vi "棋盘格搜索0元素.vi"(1 "无序一维坐标点":cluster{"X":sgl, "Y":sgl}[](array[cluster])=[{"X"=1412.6815, "Y"=3.6794338}, {"X"=950.6091, "Y"=7.2969584}, {"X"=1044.843, "Y"=8.55808}, {"X"=1048.5526, "Y"=6.4984}, {"X"=1137.2787, "Y"=6.285277}, {"X"=1139.5035, "Y"=6.383834}, {"X"=1229.4695, "Y"=6.128669}, {"X"=1233.7327, "Y"=5.9790673}, {"X"=1321.2677, "Y"=5.3170323}, {"X"=1326.042, "Y"=5.1197724}, {"X"=1418.9291, "Y"=5.099948}, {"X"=765.81134, "Y"=8.344691}, {"X"=769.6834, "Y"=8.466203}, {"X"=859.02246, "Y"=8.040275}, {"X"=862.6996, "Y"=7.9735875}, {"X"=579.4618, "Y"=10.38801}, {"X"=583.8774, "Y"=10.254913}, {"X"=950.7482, "Y"=10.59193}, {"X"=956.8515, "Y"=10.958951}, {"X"=1044.5778, "Y"=9.964842}, {"X"=1048.5502, "Y"=6.5010195}, {"X"=1137.2188, "Y"=9.72871}, {"X"=1140.8918, "Y"=9.898776}, {"X"=1229.8213, "Y"=9.607965}, {"X"=1233.8522, "Y"=9.771921}, {"X"=1321.432, "Y"=6.477976}, {"X"=1322.2452, "Y"=8.362788}, {"X"=1414.1876, "Y"=10.187137}, {"X"=1418.1567, "Y"=10.15385}, {"X"=1510.8711, "Y"=11.122694}, {"X"=394.15692, "Y"=12.698007}, {"X"=397.70276, "Y"=12.397687}, {"X"=486.81506, "Y"=11.80036}, {"X"=672.8406, "Y"=12.927005}, {"X"=676.3384, "Y"=12.897356}, {"X"=765.8697, "Y"=12.153455}, {"X"=769.6877, "Y"=11.942057}, {"X"=859.1302, "Y"=10.93324}, {"X"=209.12155, "Y"=15.971711}, {"X"=211.07715, "Y"=16.170942}, {"X"=301.63574, "Y"=15.61327}, {"X"=304.854, "Y"=17.051542}, {"X"=580.11304, "Y"=14.336995}, {"X"=583.01447, "Y"=14.092017}, {"X"=115.56893, "Y"=16.062284}, {"X"=120.1954, "Y"=17.73748}, {"X"=393.9527, "Y"=16.096884}, {"X"=397.5144, "Y"=15.868732}, {"X"=487.28784, "Y"=13.478283}, {"X"=490.1611, "Y"=13.438515}, {"X"=24.18013, "Y"=19.82086}, {"X"=28.127178, "Y"=19.778666}, {"X"=211.07715, "Y"=16.170942}, {"X"=301.23575, "Y"=17.503572}, {"X"=304.854, "Y"=17.051542}, {"X"=115.8368, "Y"=20.635664}, {"X"=120.1954, "Y"=17.73748}, {"X"=24.18013, "Y"=19.82086}, {"X"=28.127178, "Y"=19.778666}, {"X"=1045.7499, "Y"=99.26226}, {"X"=1049.2466, "Y"=98.93639}, {"X"=1138.3354, "Y"=98.90779}, {"X"=1142.3898, "Y"=98.86408}, {"X"=1231.339, "Y"=100.539635}, {"X"=1234.7195, "Y"=98.11695}, {"X"=1322.982, "Y"=98.044586}, {"X"=1327.0857, "Y"=98.04208}, {"X"=1415.0287, "Y"=97.80603}, {"X"=1419.0684, "Y"=98.0681}, {"X"=1505.3035, "Y"=96.962456}, {"X"=1512.1074, "Y"=97.130104}, {"X"=859.9964, "Y"=100.78096}, {"X"=863.6331, "Y"=100.47248}, {"X"=952.1462, "Y"=100.175026}, {"X"=957.658, "Y"=100.13256}, {"X"=580.6278, "Y"=103.213036}, {"X"=584.3985, "Y"=103.23712}, {"X"=673.80273, "Y"=102.282234}, {"X"=677.1538, "Y"=101.88441}, {"X"=767.1707, "Y"=101.07624}, {"X"=770.1185, "Y"=101.21626}, {"X"=1138.8663, "Y"=102.19401}, {"X"=1142.2152, "Y"=102.75242}, {"X"=1231.2098, "Y"=101.7738}, {"X"=1234.8201, "Y"=101.93511}, {"X"=1323.2035, "Y"=101.86018}, {"X"=1325.4602, "Y"=101.86024}, {"X"=1415.3267, "Y"=101.769135}, {"X"=1419.187, "Y"=102.09399}, {"X"=1506.1565, "Y"=102.658516}, {"X"=1508.5452, "Y"=102.83926}, {"X"=394.8409, "Y"=105.33422}, {"X"=397.97128, "Y"=106.54971}, {"X"=487.95963, "Y"=103.91474}, {"X"=489.4614, "Y"=104.11982}, {"X"=860.1312, "Y"=103.95015}, {"X"=863.5909, "Y"=103.99937}, {"X"=951.7162, "Y"=103.64365}, {"X"=957.8369, "Y"=103.65914}, {"X"=1045.9299, "Y"=102.832466}, {"X"=1049.6682, "Y"=102.73234}, {"X"=301.91907, "Y"=108.63288}, {"X"=305.55942, "Y"=106.17497}, {"X"=580.39777, "Y"=106.70424}, {"X"=673.86035, "Y"=105.7713}, {"X"=676.97003, "Y"=105.222305}, {"X"=767.33765, "Y"=105.11311}, {"X"=209.08888, "Y"=107.90821}, {"X"=213.45741, "Y"=108.1176}, {"X"=398.18994, "Y"=108.61662}, {"X"=487.44672, "Y"=107.1107}, {"X"=491.09204, "Y"=107.61974}, {"X"=584.32666, "Y"=106.886406}, {"X"=24.376457, "Y"=110.74549}, {"X"=29.008192, "Y"=112.00042}, {"X"=301.81976, "Y"=109.84095}, {"X"=305.561, "Y"=110.04465}, {"X"=117.142044, "Y"=113.09247}, {"X"=117.475876, "Y"=113.03857}, {"X"=209.28003, "Y"=111.63779}, {"X"=23.839958, "Y"=114.579}, {"X"=29.008192, "Y"=112.00042}, {"X"=1324.1991, "Y"=190.40904}, {"X"=1328.04, "Y"=190.72903}, {"X"=1415.9901, "Y"=190.3095}, {"X"=1420.0558, "Y"=189.9869}, {"X"=1507.3752, "Y"=193.75264}, {"X"=1512.9387, "Y"=189.73003}, {"X"=864.7421, "Y"=193.75208}, {"X"=952.7631, "Y"=193.2216}, {"X"=958.9441, "Y"=192.36739}, {"X"=1046.9897, "Y"=192.17368}, {"X"=1050.2294, "Y"=192.27582}, {"X"=1139.8049, "Y"=194.94722}, {"X"=1142.9745, "Y"=195.48999}, {"X"=767.46454, "Y"=194.17882}, {"X"=771.5019, "Y"=194.30862}, {"X"=861.0135, "Y"=193.35992}, {"X"=1231.742, "Y"=194.57672}, {"X"=1236.1552, "Y"=194.63904}, {"X"=1324.2634, "Y"=193.86778}, {"X"=1327.9126, "Y"=194.19914}, {"X"=1416.7396, "Y"=194.11032}, {"X"=1420.2114, "Y"=194.6422}, {"X"=1507.339, "Y"=194.16754}, {"X"=1512.0775, "Y"=194.51192}, {"X"=488.48718, "Y"=197.1191}, {"X"=491.92194, "Y"=197.1006}, {"X"=581.37964, "Y"=195.94873}, {"X"=584.89233, "Y"=195.9323}, {"X"=952.7631, "Y"=193.2216}, {"X"=958.8722, "Y"=195.93758}, {"X"=1046.9062, "Y"=195.63086}, {"X"=1050.1118, "Y"=193.37167}, {"X"=1139.8049, "Y"=194.94722}, {"X"=1142.9896, "Y"=195.51785}, {"X"=306.36182, "Y"=199.2471}, {"X"=395.10892, "Y"=197.99316}, {"X"=399.07867, "Y"=198.0709}, {"X"=678.3702, "Y"=198.62344}, {"X"=768.0162, "Y"=197.97568}, {"X"=771.06116, "Y"=198.24771}, {"X"=861.1216, "Y"=196.92929}, {"X"=864.5629, "Y"=197.49843}, {"X"=209.866, "Y"=200.47197}, {"X"=213.58813, "Y"=200.94618}, {"X"=302.78488, "Y"=198.96336}, {"X"=488.48718, "Y"=197.1191}, {"X"=492.23672, "Y"=200.02927}, {"X"=581.9015, "Y"=199.61447}, {"X"=585.0505, "Y"=199.66968}, {"X"=674.42084, "Y"=198.56363}, {"X"=25.285702, "Y"=202.90668}, {"X"=29.850668, "Y"=203.29842}, {"X"=117.47388, "Y"=204.86719}, {"X"=121.02383, "Y"=201.98978}, {"X"=306.60657, "Y"=202.69254}, {"X"=395.33936, "Y"=201.65161}, {"X"=398.54382, "Y"=201.6404}, {"X"=209.88214, "Y"=200.49939}, {"X"=213.58394, "Y"=200.949}, {"X"=25.198978, "Y"=206.81383}, {"X"=28.683458, "Y"=206.78719}, {"X"=117.47388, "Y"=204.86719}, {"X"=120.80801, "Y"=205.05066}, {"X"=1325.2671, "Y"=283.35147}, {"X"=1328.9977, "Y"=282.91864}, {"X"=1418.007, "Y"=282.4978}, {"X"=1421.0331, "Y"=282.4797}, {"X"=1509.221, "Y"=281.48706}, {"X"=1512.846, "Y"=282.29694}, {"X"=1047.7343, "Y"=285.08377}, {"X"=1051.6312, "Y"=285.14056}, {"X"=1141.0441, "Y"=284.36755}, {"X"=1144.0085, "Y"=284.42355}, {"X"=1232.844, "Y"=283.8645}, {"X"=1236.5856, "Y"=283.55615}, {"X"=768.8493, "Y"=287.1859}, {"X"=772.0435, "Y"=287.158}, {"X"=861.77344, "Y"=286.49255}, {"X"=865.5478, "Y"=286.81137}, {"X"=953.85864, "Y"=289.18365}, {"X"=959.21454, "Y"=285.9517}, {"X"=1325.3582, "Y"=286.68594}, {"X"=1329.0134, "Y"=286.73038}, {"X"=1417.3721, "Y"=286.148}, {"X"=1420.9364, "Y"=286.547}, {"X"=1509.0696, "Y"=286.48337}, {"X"=1512.7725, "Y"=286.69513}, {"X"=582.3613, "Y"=289.0204}, {"X"=586.0527, "Y"=289.16724}, {"X"=675.2951, "Y"=288.3512}, {"X"=679.0281, "Y"=287.99115}, {"X"=1047.8466, "Y"=288.6356}, {"X"=1051.0605, "Y"=289.00327}, {"X"=1140.4221, "Y"=287.8523}, {"X"=1144.0176, "Y"=287.8429}, {"X"=1236.9786, "Y"=287.531}, {"X"=396.21786, "Y"=291.33987}, {"X"=399.77203, "Y"=291.1318}, {"X"=489.97818, "Y"=290.03088}, {"X"=768.72845, "Y"=290.75858}, {"X"=862.06635, "Y"=289.9451}, {"X"=865.6694, "Y"=290.1604}, {"X"=953.85864, "Y"=289.18365}, {"X"=959.262, "Y"=289.76746}, {"X"=303.42657, "Y"=292.39053}, {"X"=306.9965, "Y"=292.31665}, {"X"=582.3937, "Y"=292.66464}, {"X"=585.84784, "Y"=292.1057}, {"X"=675.49225, "Y"=291.6714}, {"X"=678.7614, "Y"=292.08536}, {"X"=772.15295, "Y"=290.6915}, {"X"=118.36568, "Y"=294.27832}, {"X"=122.0356, "Y"=294.39282}, {"X"=396.16946, "Y"=294.61725}, {"X"=399.77203, "Y"=291.1318}, {"X"=489.8705, "Y"=294.09894}, {"X"=26.318064, "Y"=296.0619}, {"X"=29.029413, "Y"=296.98248}, {"X"=303.87878, "Y"=295.66165}, {"X"=307.0452, "Y"=295.67197}, {"X"=118.43474, "Y"=298.12512}, {"X"=121.986946, "Y"=297.7946}, {"X"=210.25739, "Y"=297.07492}, {"X"=214.33003, "Y"=296.81644}, {"X"=26.236132, "Y"=299.67172}, {"X"=29.051172, "Y"=297.44492}, {"X"=1509.8569, "Y"=375.06134}, {"X"=1515.014, "Y"=376.8497}, {"X"=1234.0524, "Y"=377.1514}, {"X"=1237.0068, "Y"=378.577}, {"X"=1326.3942, "Y"=376.00345}, {"X"=1329.9598, "Y"=375.93393}, {"X"=1418.275, "Y"=375.24207}, {"X"=1421.9374, "Y"=375.1909}, {"X"=954.8097, "Y"=378.36212}, {"X"=960.02106, "Y"=378.7047}, {"X"=1048.6476, "Y"=377.7871}, {"X"=1052.6216, "Y"=381.06326}, {"X"=1141.4268, "Y"=377.3096}, {"X"=1144.7307, "Y"=377.1711}, {"X"=1509.8569, "Y"=375.06134}, {"X"=1515.014, "Y"=376.8497}, {"X"=676.14905, "Y"=381.02945}, {"X"=769.40826, "Y"=380.4111}, {"X"=773.4843, "Y"=382.63983}, {"X"=862.42065, "Y"=379.4066}, {"X"=866.0779, "Y"=379.43088}, {"X"=1234.1095, "Y"=380.14008}, {"X"=1237.6244, "Y"=380.54337}, {"X"=1326.2516, "Y"=379.63504}, {"X"=1329.8422, "Y"=379.65314}, {"X"=1418.265, "Y"=378.85614}, {"X"=1421.9978, "Y"=379.1067}, {"X"=489.97784, "Y"=383.07867}, {"X"=493.81558, "Y"=382.8947}, {"X"=583.03766, "Y"=382.16656}, {"X"=586.826, "Y"=381.96048}, {"X"=954.73126, "Y"=382.2282}, {"X"=960.02106, "Y"=378.7047}, {"X"=1048.79, "Y"=381.73087}, {"X"=1052.6216, "Y"=381.06326}, {"X"=304.3866, "Y"=384.95547}, {"X"=307.9497, "Y"=385.10504}, {"X"=400.6453, "Y"=386.56058}, {"X"=676.1419, "Y"=384.64987}, {"X"=680.2898, "Y"=384.6469}, {"X"=769.6665, "Y"=383.59375}, {"X"=773.4509, "Y"=383.54562}, {"X"=862.7106, "Y"=383.15347}, {"X"=865.9845, "Y"=383.1695}, {"X"=122.703026, "Y"=387.3263}, {"X"=212.04758, "Y"=386.27716}, {"X"=215.01054, "Y"=386.17075}, {"X"=490.1799, "Y"=386.67773}, {"X"=493.9983, "Y"=386.97186}, {"X"=582.9337, "Y"=385.84512}, {"X"=587.5356, "Y"=385.06296}, {"X"=27.18197, "Y"=388.38385}, {"X"=27.18197, "Y"=388.38385}, {"X"=397.07806, "Y"=387.55035}, {"X"=211.91324, "Y"=389.84753}, {"X"=215.16852, "Y"=389.67154}, {"X"=26.72049, "Y"=391.7773}, {"X"=30.596046, "Y"=392.024}, {"X"=209.9042, "Y"=399.12137}, {"X"=1327.3544, "Y"=469.0647}, {"X"=1419.2324, "Y"=468.16718}, {"X"=1510.364, "Y"=467.17642}, {"X"=1514.4918, "Y"=470.6456}, {"X"=1049.9957, "Y"=471.0501}, {"X"=1052.8948, "Y"=470.93842}, {"X"=1142.4253, "Y"=470.17645}, {"X"=1145.9662, "Y"=470.30652}, {"X"=1235.0592, "Y"=469.96625}, {"X"=1238.565, "Y"=469.9739}, {"X"=864.0924, "Y"=472.51093}, {"X"=866.97833, "Y"=472.8782}, {"X"=955.69977, "Y"=471.45383}, {"X"=961.07306, "Y"=471.75146}, {"X"=1327.6859, "Y"=472.58783}, {"X"=1330.6233, "Y"=471.96988}, {"X"=1419.2172, "Y"=471.65576}, {"X"=1514.5454, "Y"=471.04782}, {"X"=680.64746, "Y"=474.37677}, {"X"=770.34247, "Y"=473.3417}, {"X"=774.00336, "Y"=473.83273}, {"X"=1049.3457, "Y"=474.62115}, {"X"=1142.9866, "Y"=473.95023}, {"X"=1145.7654, "Y"=473.9458}, {"X"=1234.9541, "Y"=473.04596}, {"X"=397.9174, "Y"=477.19165}, {"X"=402.21198, "Y"=477.09775}, {"X"=494.78082, "Y"=475.7434}, {"X"=584.2983, "Y"=474.8645}, {"X"=587.1738, "Y"=475.39746}, {"X"=864.05634, "Y"=476.47598}, {"X"=866.8885, "Y"=476.4903}, {"X"=955.8802, "Y"=475.2065}, {"X"=961.29596, "Y"=475.23154}, {"X"=212.9732, "Y"=479.274}, {"X"=216.23286, "Y"=479.20996}, {"X"=305.33755, "Y"=478.36325}, {"X"=308.86752, "Y"=478.19977}, {"X"=680.756, "Y"=477.63123}, {"X"=769.9319, "Y"=476.64694}, {"X"=773.70013, "Y"=476.8528}, {"X"=120.21636, "Y"=480.98227}, {"X"=123.844246, "Y"=480.48163}, {"X"=398.3618, "Y"=480.89243}, {"X"=401.6019, "Y"=480.75598}, {"X"=491.27213, "Y"=479.9286}, {"X"=494.78894, "Y"=479.69577}, {"X"=584.1824, "Y"=478.77087}, {"X"=587.6954, "Y"=478.91016}, {"X"=674.01056, "Y"=482.62982}, {"X"=212.80879, "Y"=482.5869}, {"X"=216.24107, "Y"=482.4923}, {"X"=305.47998, "Y"=481.54013}, {"X"=308.94867, "Y"=481.53357}, {"X"=31.690287, "Y"=484.7523}, {"X"=120.27868, "Y"=483.6429}, {"X"=123.6863, "Y"=483.62024}, {"X"=28.121384, "Y"=484.84103}, {"X"=1420.168, "Y"=559.44476}, {"X"=1423.1482, "Y"=559.8198}, {"X"=1511.3728, "Y"=558.7311}, {"X"=1514.719, "Y"=558.60486}, {"X"=1235.4536, "Y"=561.34454}, {"X"=1239.2461, "Y"=561.0861}, {"X"=1327.4503, "Y"=560.7745}, {"X"=1331.5977, "Y"=560.3296}, {"X"=1050.0205, "Y"=562.883}, {"X"=1053.6465, "Y"=563.0215}, {"X"=1142.638, "Y"=561.9079}, {"X"=1146.5131, "Y"=562.1473}, {"X"=772.0103, "Y"=565.13245}, {"X"=864.98785, "Y"=564.5342}, {"X"=864.98785, "Y"=564.5342}, {"X"=956.3751, "Y"=563.2659}, {"X"=962.3416, "Y"=563.8341}, {"X"=1511.809, "Y"=564.7066}, {"X"=588.1273, "Y"=567.27527}, {"X"=677.9531, "Y"=566.30536}, {"X"=681.8815, "Y"=565.8051}, {"X"=1329.0206, "Y"=566.27405}, {"X"=1329.0206, "Y"=566.27405}, {"X"=1420.063, "Y"=565.6257}, {"X"=1423.6278, "Y"=565.2837}, {"X"=1515.6139, "Y"=564.82184}, {"X"=396.0596, "Y"=569.9061}, {"X"=492.20886, "Y"=567.94684}, {"X"=495.66125, "Y"=568.28503}, {"X"=1050.3988, "Y"=568.6675}, {"X"=1053.7635, "Y"=568.8372}, {"X"=1143.1594, "Y"=567.572}, {"X"=1235.687, "Y"=567.51605}, {"X"=1239.5625, "Y"=566.922}, {"X"=213.8178, "Y"=570.6908}, {"X"=217.59773, "Y"=571.0198}, {"X"=306.02786, "Y"=570.01575}, {"X"=310.0028, "Y"=569.8299}, {"X"=864.40247, "Y"=570.1614}, {"X"=956.572, "Y"=569.1915}, {"X"=962.70074, "Y"=568.88965}, {"X"=32.6733, "Y"=572.6269}, {"X"=121.22974, "Y"=571.9324}, {"X"=678.23785, "Y"=572.22437}, {"X"=682.0419, "Y"=572.0976}, {"X"=771.42706, "Y"=571.2061}, {"X"=868.0665, "Y"=570.3193}, {"X"=492.17953, "Y"=573.8406}, {"X"=496.0425, "Y"=573.9344}, {"X"=588.7999, "Y"=572.8369}, {"X"=306.35614, "Y"=575.8801}, {"X"=309.8908, "Y"=575.51245}, {"X"=399.4254, "Y"=575.22363}, {"X"=121.18887, "Y"=577.85657}, {"X"=213.71536, "Y"=576.2731}, {"X"=217.2551, "Y"=576.7435}, {"X"=29.451935, "Y"=578.9594}, {"X"=1424.0056, "Y"=652.84735}, {"X"=1512.0708, "Y"=652.91266}, {"X"=1515.6927, "Y"=652.30774}, {"X"=1236.1508, "Y"=655.2158}, {"X"=1239.8197, "Y"=655.1497}, {"X"=1328.7433, "Y"=654.4055}, {"X"=1331.8887, "Y"=654.169}, {"X"=1420.2484, "Y"=653.17346}, {"X"=1051.1462, "Y"=657.3596}, {"X"=1054.7452, "Y"=657.3702}, {"X"=1143.0564, "Y"=657.12195}, {"X"=1147.328, "Y"=656.19324}, {"X"=1512.3021, "Y"=656.55066}, {"X"=1512.4271, "Y"=656.50757}, {"X"=868.06213, "Y"=658.3889}, {"X"=957.827, "Y"=658.16974}, {"X"=962.7932, "Y"=658.1109}, {"X"=1236.2236, "Y"=658.6412}, {"X"=1239.5663, "Y"=658.8228}, {"X"=1328.7885, "Y"=657.8645}, {"X"=1331.859, "Y"=657.7278}, {"X"=1423.7322, "Y"=657.41034}, {"X"=679.29376, "Y"=660.33417}, {"X"=772.2044, "Y"=662.99475}, {"X"=775.7194, "Y"=659.479}, {"X"=1051.1462, "Y"=657.3596}, {"X"=1054.7452, "Y"=657.3702}, {"X"=1142.9763, "Y"=657.51434}, {"X"=1147.4087, "Y"=659.037}, {"X"=493.21652, "Y"=662.3159}, {"X"=496.71637, "Y"=662.33325}, {"X"=589.6308, "Y"=661.3398}, {"X"=868.8922, "Y"=661.8618}, {"X"=957.336, "Y"=661.77264}, {"X"=961.2878, "Y"=663.0072}, {"X"=215.13858, "Y"=664.4556}, {"X"=217.96014, "Y"=664.7446}, {"X"=307.19785, "Y"=663.9552}, {"X"=311.07373, "Y"=664.37274}, {"X"=400.31244, "Y"=663.33}, {"X"=404.0007, "Y"=663.2761}, {"X"=586.37366, "Y"=665.0964}, {"X"=682.7313, "Y"=663.8328}, {"X"=772.2044, "Y"=662.99475}, {"X"=775.2198, "Y"=663.5096}, {"X"=30.386137, "Y"=666.41254}, {"X"=33.78909, "Y"=666.9363}, {"X"=122.40613, "Y"=665.84503}, {"X"=126.02608, "Y"=665.8279}, {"X"=492.90775, "Y"=665.8436}, {"X"=496.92422, "Y"=665.8403}, {"X"=214.90646, "Y"=668.46643}, {"X"=218.53204, "Y"=668.5923}, {"X"=307.47598, "Y"=667.53406}, {"X"=311.1581, "Y"=667.7079}, {"X"=403.96774, "Y"=666.58673}, {"X"=30.956583, "Y"=670.09735}, {"X"=31.453695, "Y"=670.0807}, {"X"=122.94276, "Y"=669.6548}, {"X"=125.77965, "Y"=669.294}, {"X"=1512.6708, "Y"=744.44354}, {"X"=1516.6038, "Y"=744.8743}, {"X"=1332.8044, "Y"=746.6566}, {"X"=1421.0765, "Y"=745.85065}, {"X"=1424.6377, "Y"=749.5571}, {"X"=1145.8118, "Y"=748.033}, {"X"=1146.9818, "Y"=748.2303}, {"X"=1236.9733, "Y"=748.09424}, {"X"=1236.9733, "Y"=748.09424}, {"X"=1512.4379, "Y"=748.0738}, {"X"=1516.5994, "Y"=748.53796}, {"X"=957.71515, "Y"=751.041}, {"X"=963.9972, "Y"=751.08954}, {"X"=1051.8019, "Y"=749.85675}, {"X"=1055.163, "Y"=749.92584}, {"X"=1332.627, "Y"=750.5142}, {"X"=1420.7009, "Y"=749.6165}, {"X"=1424.658, "Y"=749.5828}, {"X"=773.14355, "Y"=752.3674}, {"X"=866.12976, "Y"=751.4759}, {"X"=868.864, "Y"=754.5674}, {"X"=1144.3915, "Y"=752.5427}, {"X"=1147.6367, "Y"=752.30023}, {"X"=1237.0159, "Y"=751.5042}, {"X"=494.73883, "Y"=755.6712}, {"X"=497.8763, "Y"=755.1298}, {"X"=587.28986, "Y"=754.1544}, {"X"=679.9945, "Y"=753.2988}, {"X"=683.91077, "Y"=753.28455}, {"X"=957.874, "Y"=752.513}, {"X"=963.9972, "Y"=751.08954}, {"X"=1051.715, "Y"=752.9354}, {"X"=1055.2142, "Y"=753.10297}, {"X"=308.51486, "Y"=756.83453}, {"X"=311.88177, "Y"=756.9832}, {"X"=404.83005, "Y"=755.91406}, {"X"=772.84546, "Y"=755.67035}, {"X"=776.7339, "Y"=756.0081}, {"X"=868.2573, "Y"=755.0738}, {"X"=31.860968, "Y"=759.42645}, {"X"=35.618187, "Y"=759.91064}, {"X"=123.8723, "Y"=758.613}, {"X"=125.50653, "Y"=758.1765}, {"X"=216.27132, "Y"=757.9219}, {"X"=219.32713, "Y"=757.7127}, {"X"=497.8763, "Y"=755.1298}, {"X"=587.0371, "Y"=757.8683}, {"X"=590.6328, "Y"=757.74884}, {"X"=680.9836, "Y"=757.37994}, {"X"=309.1065, "Y"=760.28265}, {"X"=312.00598, "Y"=760.57916}, {"X"=404.73682, "Y"=759.76105}, {"X"=494.2343, "Y"=759.09515}, {"X"=1053.7183, "Y"=759.52075}, {"X"=32.036686, "Y"=762.72076}, {"X"=123.82045, "Y"=762.20496}, {"X"=127.40294, "Y"=762.11786}, {"X"=216.3088, "Y"=761.10406}, {"X"=219.51328, "Y"=760.9907}, {"X"=1512.7866, "Y"=836.7208}, {"X"=1516.1836, "Y"=836.706}, {"X"=1421.265, "Y"=838.0971}, {"X"=1237.2886, "Y"=840.30884}, {"X"=1240.8717, "Y"=840.2423}, {"X"=1516.0099, "Y"=840.84064}, {"X"=1052.3063, "Y"=842.35706}, {"X"=1055.8276, "Y"=842.0459}, {"X"=1144.8585, "Y"=841.3377}, {"X"=1421.244, "Y"=842.0497}, {"X"=775.316, "Y"=845.4439}, {"X"=866.7553, "Y"=843.96124}, {"X"=870.1111, "Y"=844.3156}, {"X"=966.4094, "Y"=845.16437}, {"X"=1148.0193, "Y"=844.9224}, {"X"=1237.1177, "Y"=843.7787}, {"X"=1240.814, "Y"=843.8384}, {"X"=1329.8593, "Y"=842.6638}, {"X"=1333.1106, "Y"=842.70825}, {"X"=588.2757, "Y"=846.72455}, {"X"=591.5033, "Y"=847.0653}, {"X"=681.00464, "Y"=846.18243}, {"X"=685.01025, "Y"=846.3228}, {"X"=774.0265, "Y"=845.37006}, {"X"=1052.2452, "Y"=845.84656}, {"X"=1055.5713, "Y"=845.9697}, {"X"=402.46408, "Y"=848.4553}, {"X"=405.85208, "Y"=849.1168}, {"X"=494.95795, "Y"=848.1302}, {"X"=498.768, "Y"=848.0817}, {"X"=863.88965, "Y"=845.8309}, {"X"=870.37415, "Y"=844.3211}, {"X"=958.74976, "Y"=846.77563}, {"X"=125.33506, "Y"=850.9014}, {"X"=128.75377, "Y"=851.14294}, {"X"=217.27446, "Y"=850.38837}, {"X"=309.9121, "Y"=849.8526}, {"X"=313.24408, "Y"=852.8987}, {"X"=587.80383, "Y"=850.5033}, {"X"=591.61615, "Y"=850.7564}, {"X"=681.3442, "Y"=849.82886}, {"X"=684.9827, "Y"=847.42126}, {"X"=33.159054, "Y"=852.04767}, {"X"=402.47308, "Y"=852.20996}, {"X"=405.83694, "Y"=852.06805}, {"X"=495.41132, "Y"=851.6362}, {"X"=498.69678, "Y"=851.55646}, {"X"=125.36255, "Y"=854.8094}, {"X"=128.62521, "Y"=853.93445}, {"X"=217.24501, "Y"=853.59094}, {"X"=221.00249, "Y"=854.06195}, {"X"=309.84454, "Y"=852.7346}, {"X"=313.24408, "Y"=852.8987}, {"X"=33.18453, "Y"=853.3919}, {"X"=1094.8916, "Y"=879.7679}, {"X"=1326.8314, "Y"=920.89703}, {"X"=1324.2201, "Y"=923.777}, {"X"=1325.2799, "Y"=923.7304}, {"X"=1513.0775, "Y"=929.07574}, {"X"=1516.8359, "Y"=928.95483}, {"X"=1421.9668, "Y"=930.1851}, {"X"=1425.1039, "Y"=930.08386}, {"X"=1237.4916, "Y"=933.0584}, {"X"=1240.8352, "Y"=932.4593}, {"X"=1331.0498, "Y"=931.4504}, {"X"=1331.0498, "Y"=931.4504}, {"X"=1512.8682, "Y"=932.8561}, {"X"=1516.886, "Y"=932.69073}, {"X"=1053.2501, "Y"=934.4577}, {"X"=1053.2501, "Y"=934.4577}, {"X"=1145.7811, "Y"=934.0479}, {"X"=1149.4984, "Y"=933.73804}, {"X"=1421.3748, "Y"=933.98804}, {"X"=1424.8423, "Y"=934.2104}, {"X"=867.4395, "Y"=937.1504}, {"X"=870.9637, "Y"=936.9113}, {"X"=959.7388, "Y"=935.8997}, {"X"=965.13367, "Y"=935.7838}, {"X"=1237.4745, "Y"=935.89185}, {"X"=1241.134, "Y"=935.9662}, {"X"=1330.0884, "Y"=934.9351}, {"X"=1333.5903, "Y"=935.0333}, {"X"=682.15985, "Y"=938.4487}, {"X"=685.06586, "Y"=938.4208}, {"X"=774.95917, "Y"=938.17334}, {"X"=778.5676, "Y"=938.227}, {"X"=1053.1005, "Y"=937.9979}, {"X"=1056.5786, "Y"=937.8953}, {"X"=1145.3656, "Y"=937.22943}, {"X"=1148.7098, "Y"=937.257}, {"X"=403.44504, "Y"=941.33777}, {"X"=406.92322, "Y"=940.8044}, {"X"=496.3331, "Y"=941.0075}, {"X"=499.9358, "Y"=940.97577}, {"X"=589.3127, "Y"=939.8238}, {"X"=867.4395, "Y"=937.1504}, {"X"=870.9637, "Y"=936.9113}, {"X"=959.3603, "Y"=939.2864}, {"X"=965.25543, "Y"=939.3708}, {"X"=222.5551, "Y"=942.39026}, {"X"=311.01688, "Y"=942.26483}, {"X"=314.80524, "Y"=943.13434}, {"X"=682.1386, "Y"=942.0657}, {"X"=685.58167, "Y"=942.0178}, {"X"=775.2412, "Y"=939.3993}, {"X"=778.5166, "Y"=941.0647}, {"X"=34.832672, "Y"=943.8151}, {"X"=34.832672, "Y"=943.8151}, {"X"=126.3559, "Y"=943.4925}, {"X"=130.02597, "Y"=943.2728}, {"X"=496.45908, "Y"=944.1266}, {"X"=499.9358, "Y"=940.97577}, {"X"=589.3983, "Y"=943.6146}, {"X"=592.84216, "Y"=941.2381}, {"X"=218.91013, "Y"=946.0248}, {"X"=222.81172, "Y"=945.8305}, {"X"=311.21887, "Y"=945.63025}, {"X"=314.0045, "Y"=945.7016}, {"X"=403.43817, "Y"=944.6669}, {"X"=407.33734, "Y"=944.66846}, {"X"=34.753956, "Y"=947.16754}, {"X"=37.952045, "Y"=945.3175}, {"X"=1513.1074, "Y"=1020.53687}, {"X"=1516.7944, "Y"=1020.3726}, {"X"=1422.1199, "Y"=1022.3085}, {"X"=1422.4272, "Y"=1022.35815}, {"X"=1237.7603, "Y"=1025.2195}, {"X"=1241.5918, "Y"=1024.5043}, {"X"=1330.0405, "Y"=1023.4761}, {"X"=1333.5803, "Y"=1023.4029}, {"X"=1512.2899, "Y"=1024.6274}, {"X"=1516.7074, "Y"=1024.4958}, {"X"=1053.4192, "Y"=1027.228}, {"X"=1057.2833, "Y"=1027.4166}, {"X"=1146.0155, "Y"=1026.057}, {"X"=1149.5197, "Y"=1026.0944}, {"X"=1422.1165, "Y"=1025.9506}, {"X"=1425.0371, "Y"=1025.8577}, {"X"=871.8444, "Y"=1029.0967}, {"X"=959.8629, "Y"=1027.9442}, {"X"=965.6788, "Y"=1027.915}, {"X"=1237.7603, "Y"=1025.2195}, {"X"=1241.622, "Y"=1028.4213}, {"X"=1330.1205, "Y"=1026.9482}, {"X"=1333.6062, "Y"=1027.1625}, {"X"=682.9343, "Y"=1031.4572}, {"X"=686.32434, "Y"=1030.9644}, {"X"=775.43744, "Y"=1030.3405}, {"X"=779.281, "Y"=1030.3405}, {"X"=868.21136, "Y"=1029.3007}, {"X"=1053.4773, "Y"=1030.0444}, {"X"=1057.2833, "Y"=1027.4166}, {"X"=1146.203, "Y"=1029.6053}, {"X"=1149.5355, "Y"=1026.4617}, {"X"=497.30618, "Y"=1033.2229}, {"X"=500.91095, "Y"=1033.2767}, {"X"=590.36127, "Y"=1032.0253}, {"X"=593.9072, "Y"=1031.889}, {"X"=959.7527, "Y"=1031.7665}, {"X"=966.0734, "Y"=1031.222}, {"X"=220.08049, "Y"=1035.1736}, {"X"=223.77623, "Y"=1035.241}, {"X"=312.41544, "Y"=1034.2931}, {"X"=315.8206, "Y"=1034.3982}, {"X"=405.34964, "Y"=1033.7988}, {"X"=408.60822, "Y"=1033.7543}, {"X"=682.841, "Y"=1034.1649}, {"X"=682.841, "Y"=1034.1649}, {"X"=776.06824, "Y"=1033.6057}, {"X"=778.93896, "Y"=1033.6743}, {"X"=868.1692, "Y"=1032.6964}, {"X"=872.0014, "Y"=1032.8055}, {"X"=36.842037, "Y"=1035.9076}, {"X"=39.936604, "Y"=1035.942}, {"X"=128.4923, "Y"=1035.3223}, {"X"=131.72397, "Y"=1035.3107}, {"X"=497.30618, "Y"=1033.2229}, {"X"=501.04752, "Y"=1036.593}, {"X"=589.87683, "Y"=1035.6193}, {"X"=593.91644, "Y"=1035.6195}, {"X"=220.08049, "Y"=1035.1736}, {"X"=223.65102, "Y"=1038.0187}, {"X"=312.88974, "Y"=1037.5582}, {"X"=315.66324, "Y"=1035.3694}, {"X"=405.17947, "Y"=1037.0765}, {"X"=36.871353, "Y"=1039.5012}, {"X"=40.06816, "Y"=1039.0924}, {"X"=128.34323, "Y"=1039.046}, {"X"=131.75531, "Y"=1039.057}, {"X"=313.3858, "Y"=1095.004}, {"X"=316.9034, "Y"=1099.374}, {"X"=1517.0452, "Y"=1112.1788}, {"X"=1330.4326, "Y"=1115.1825}, {"X"=1333.8274, "Y"=1115.1122}, {"X"=1421.7859, "Y"=1113.9792}, {"X"=1425.6499, "Y"=1113.939}, {"X"=1238.3629, "Y"=1116.9702}, {"X"=1242.0442, "Y"=1116.4863}, {"X"=1513.075, "Y"=1116.5619}, {"X"=1516.7253, "Y"=1116.6143}, {"X"=1053.9915, "Y"=1119.3153}, {"X"=1057.8392, "Y"=1119.2094}, {"X"=1146.4037, "Y"=1117.9922}, {"X"=1149.7257, "Y"=1118.2214}, {"X"=1421.878, "Y"=1117.6423}, {"X"=1425.1816, "Y"=1117.8027}, {"X"=960.61615, "Y"=1120.3813}, {"X"=966.5916, "Y"=1123.5236}, {"X"=1238.2561, "Y"=1119.9944}, {"X"=1241.798, "Y"=1120.231}, {"X"=777.1195, "Y"=1122.3763}, {"X"=779.82605, "Y"=1122.7509}, {"X"=869.13324, "Y"=1124.7325}, {"X"=1053.9915, "Y"=1119.3153}, {"X"=1057.8392, "Y"=1119.2094}, {"X"=1146.2975, "Y"=1121.5195}, {"X"=1149.6943, "Y"=1121.6158}, {"X"=498.38565, "Y"=1125.3086}, {"X"=502.0334, "Y"=1125.106}, {"X"=591.2226, "Y"=1124.0642}, {"X"=594.78864, "Y"=1123.7322}, {"X"=684.0514, "Y"=1126.7501}, {"X"=960.99854, "Y"=1123.7999}, {"X"=966.5531, "Y"=1123.76}, {"X"=130.10886, "Y"=1127.1348}, {"X"=133.22865, "Y"=1127.1709}, {"X"=221.75378, "Y"=1127.1466}, {"X"=225.48451, "Y"=1127.055}, {"X"=313.80075, "Y"=1126.9071}, {"X"=317.21503, "Y"=1126.3654}, {"X"=406.46625, "Y"=1128.915}, {"X"=409.8158, "Y"=1129.1194}, {"X"=687.5572, "Y"=1127.0116}, {"X"=776.7782, "Y"=1125.7067}, {"X"=780.0457, "Y"=1125.8667}, {"X"=869.13324, "Y"=1124.7325}, {"X"=37.945602, "Y"=1127.3896}, {"X"=41.87246, "Y"=1127.2628}, {"X"=499.2134, "Y"=1128.6807}, {"X"=502.0334, "Y"=1125.106}, {"X"=591.24805, "Y"=1127.5718}, {"X"=594.9117, "Y"=1127.5956}, {"X"=221.83293, "Y"=1130.5206}, {"X"=225.48451, "Y"=1127.055}, {"X"=313.7707, "Y"=1129.5864}, {"X"=317.70578, "Y"=1129.7416}, {"X"=406.46625, "Y"=1128.915}, {"X"=409.8158, "Y"=1129.1194}, {"X"=38.267227, "Y"=1131.0507}, {"X"=41.550556, "Y"=1131.6764}, {"X"=133.1631, "Y"=1130.7614}]) -> (0 "数值输入控件":i32)   [LabVIEW 2014]
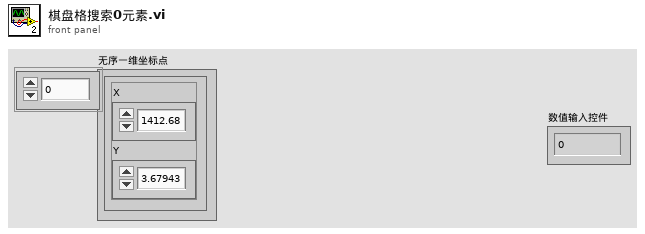
[diagram p1: front panel]
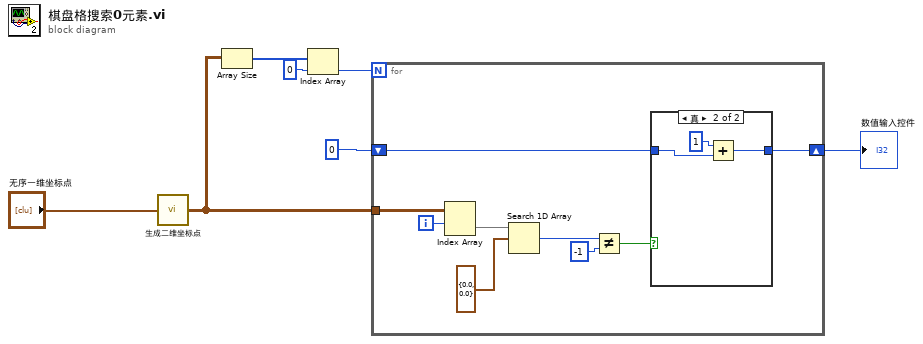
[diagram p0: block diagram]
diagram:
  n1 = call "生成二维坐标点.vi"("输入无序一维坐标点"="无序一维坐标点") -> ("输出有序二维坐标点"=w7:cluster{"X":sgl, "Y":sgl}[][])
  n2 = Array Size(array=w7) -> (size(s)=w6:i32[])
  n3 = Index Array(array=w6, index=0 ("索引")) -> (element=w4:i32)
  n4 = for {
    N: w4 -> [_]
    tunnel: w7 -> [w16]
    shift-right: [w12] -> w2
    shift-left: 0 -> [w11]
    i -> [w15]
    n5 = Index Array(array=w16, index (row)=w15) -> (element=w14:cluster{"X":sgl, "Y":sgl}[])  [unwired: 1 in]
    n6 = Search 1D Array(1D array=w14, element=cluster{"X":sgl, "Y":sgl} {"X"=0.0, "Y"=0.0} ("元素")) -> (index of element=w10:i32)  [unwired: 1 in]
    n7 = Not Equal?(x=w10, y=-1) -> (x != y?=w8:bool)
    n8 = case shown="真" w8 {
      tunnel: [w17 w20] -> w12
      tunnel: w11 -> [w17 w19]
      frame False {
      }
      frame True {
        n9 = Add(x=1, y=w19) -> (x+y=w20:i32)
      }
    }
  }
  "数值输入控件" <- w2
